vi "Extract Varint Bytes.vi"(11 "Buffer in":u8[](array[numeric]) format="%.0x") -> (2 "Varint Bytes":u8[](array[numeric]) format="%.0x", 3 "Buffer":u8[](array[numeric]) format="%.0x")   [LabVIEW 2020, in "LV-Proto.lvlib"]
uses:
  LV-Proto.lvlib
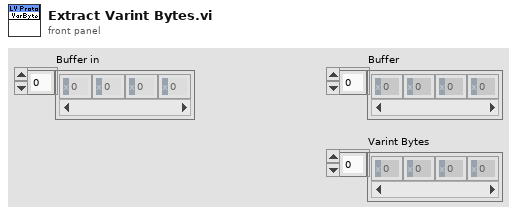
[diagram p1: front panel]
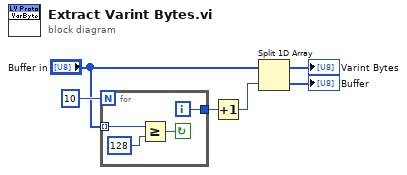
[diagram p0: block diagram]
diagram:
  n1 = for {
    N: 10 -> [_]
    tunnel: "Buffer in" -> [w10] mode=indexing
    tunnel: [w7] -> w5
    i -> [w7]
    stop <- w8 continue-if-true
    n2 = Greater Or Equal?(x=w10, y=u8 128) -> (x >= y?=w8:bool)
  }
  n3 = Increment(x=w5) -> (x+1=w4:i32)
  n4 = Split 1D Array(array="Buffer in", index=w4) -> (first subarray=→"Varint Bytes":u8[], second subarray=→"Buffer":u8[])
